vi "Swerve Drive.vi"(0 "X":dbl format="%#_13g", 1 "Z":dbl format="%#_13g", 3 "error in":errorcluster, 5 "Y":dbl format="%#_13g", 6 "Swerve Dev Ref":T3[](array[typedef]), 8 "Drive Dev Ref":T3[](array[typedef]), 9 "Straight Drive":bool, 10 "PigeonIMUDevRef":T1={"DeviceStatus"={"status"=FALSE, "code"=0, "source"=""}, "Device Number"=0, "Type"=352321536, "Device ID"=0, "Handle"=0, "UsageFrame"=0, "Library Path"=path ""} {"Type" items=["CAN"=352321536, "TalonSRX"=33554432]}, 11 "Reverse Drive":bool, 12 "Low Sensitivity":bool, 14 "X Drive":bool, 15 "Field Relative Active":bool) -> (4 "error out":errorcluster)   [LabVIEW 2017, in "Huskie Swerve.lvlib"]
uses:
  Huskie Swerve.lvlib
  <vilib>/Rock Robotics/WPI/MotorControl/WPI_MotorControlDeviceRef.ctl
  <vilib>/Rock Robotics/WPI/MotorControl/WPI_MotorControlType.ctl
  <vilib>/Rock Robotics/SystemInterfaces/DIO/FPGA_DIOPWMChannel.ctl
  <vilib>/Rock Robotics/WPI/PWM/WPI_PWMDeadband.ctl
  <vilib>/Rock Robotics/SystemInterfaces/DIO/FPGA_DIOChannel.ctl
  <vilib>/Rock Robotics/WPI/ThirdParty/Phoenix-LabVIEW/Pigeon IMU/CTRE_PigeonIMU_DeviceRef.ctl
  Public/Documents/Cross The Road Electronics/Phoenix-LabVIEW/Pigeon IMU/CTRE_PigeonIMU_ConnectionType.ctl
  <vilib>/Rock Robotics/WPI/ThirdParty/Phoenix-LabVIEW/Motor Controller/Controls/CTRE_Phoenix_MotorControl_ControlMode.ctl
panel:
  out "Constants":cluster{"a":dbl, "b":dbl, "c":dbl, "d":dbl}[](array[cluster])
  out "Direction":dbl[](array[numeric])
  out "current pos":dbl[](array[numeric])
  out "setpoint":dbl[](array[numeric])
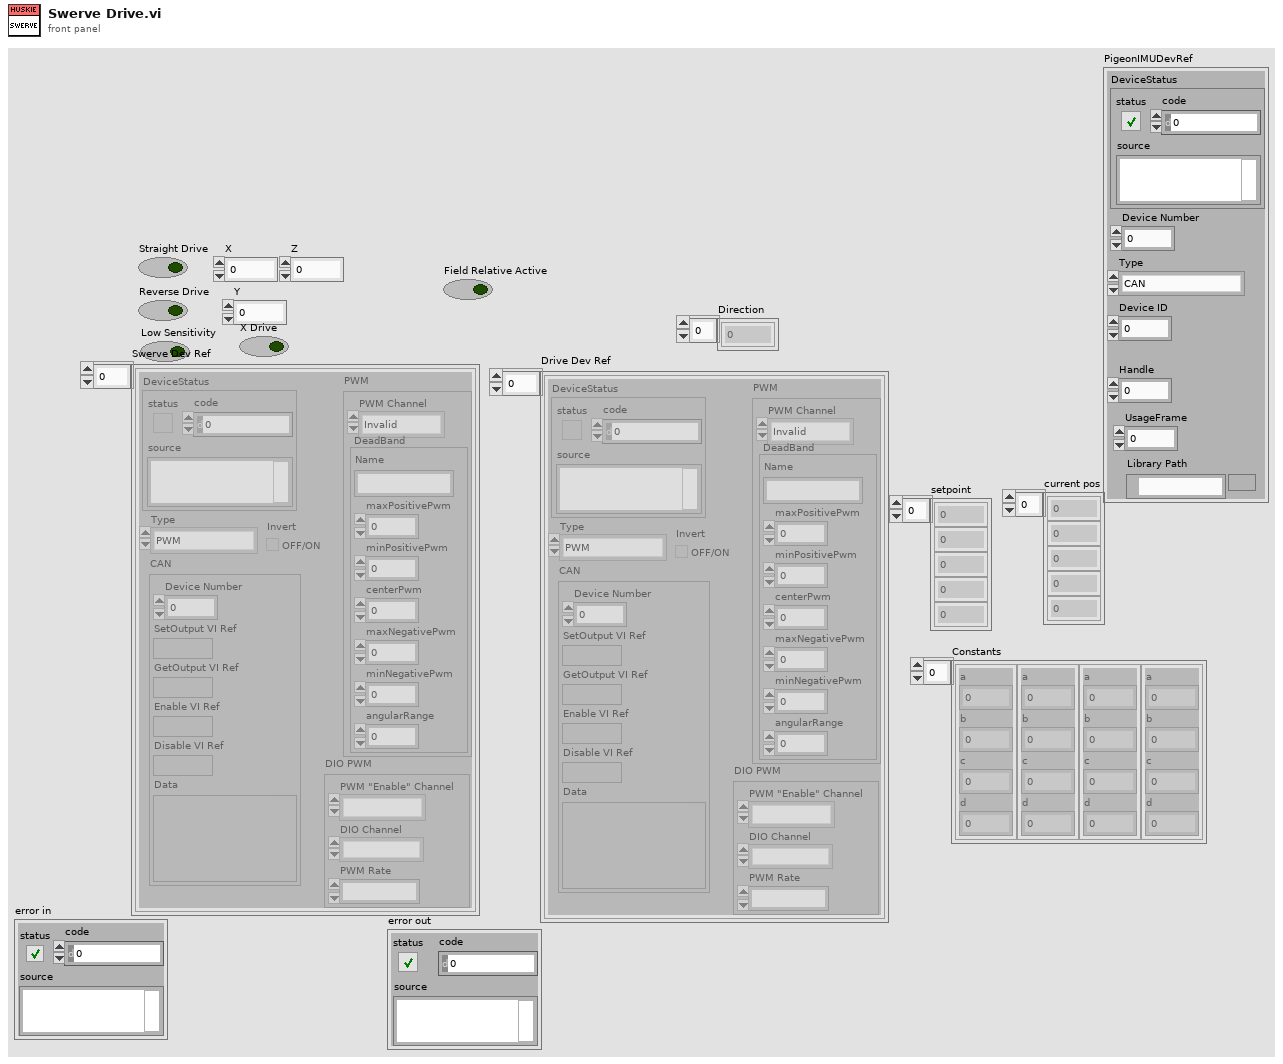
[diagram p1: front panel]
types:
  T1 = typedef "CTRE_PigeonIMU_DeviceRef.ctl" = cluster{"DeviceStatus":errorcluster, "Device Number":u8, "Type":T2, "Device ID":u32, "Handle":u64, "UsageFrame":u32, "Library Path":path}
  T2 = typedef "CTRE_PigeonIMU_ConnectionType.ctl" = u32
  T3 = typedef "WPI_MotorControlDeviceRef.ctl" = cluster{"DeviceStatus":errorcluster, "Type":T4, "PWM":cluster{"PWM Channel":T5, "DeadBand":T6}, "CAN":cluster{"Device Number":u8, "SetOutput VI Ref":variant, "GetOutput VI Ref":variant, "Enable VI Ref":variant, "Disable VI Ref":variant, "Data":variant}, "Invert":bool, "DIO PWM":cluster{"PWM \"Enable\" Channel":T5, "DIOChannel":T7, "PWM Rate":dbl}}
  T4 = typedef "WPI_MotorControlType.ctl" = enum16{"PWM", "CAN", "DIO PWM"}
  T5 = typedef "FPGA_DIOPWMChannel.ctl" = enum8{"PWM 0", "PWM 1", "PWM 2", "PWM 3", "PWM 4", "PWM 5", "PWM 6", "PWM 7", "PWM 8", "PWM 9", "PWM MXP 0", "PWM MXP 1", "PWM MXP 2", "PWM MXP 3", "PWM MXP 4", "PWM MXP 5", "PWM MXP 6", "PWM MXP 7", "PWM MXP 8", "PWM MXP 9", "Invalid"}
  T6 = typedef "WPI_PWMDeadband.ctl" = cluster{"Name":string, "maxPositivePwm":i32, "minPositivePwm":i32, "centerPwm":i32, "maxNegativePwm":i32, "minNegativePwm":i32, "angularRange":u16}
  T7 = typedef "FPGA_DIOChannel.ctl" = enum8{"DIO 0", "DIO 1", "DIO 2", "DIO 3", "DIO 4", "DIO 5", "DIO 6", "DIO 7", "DIO 8", "DIO 9", "DIO MXP 0", "DIO MXP 1", "DIO MXP 2", "DIO MXP 3", "DIO MXP 4", "DIO MXP 5", "DIO MXP 6", "DIO MXP 7", "DIO MXP 8", "DIO MXP 9", "DIO MXP 10", "DIO MXP 11", "DIO MXP 12", "DIO MXP 13", "DIO MXP 14", "DIO MXP 15", "SPI Port CS1", "SPI Port CS2", "SPI Port CS3", "SPI Port MISO", "SPI Port MOSI", "Invalid"}
  T8 = typedef "CTRE_Phoenix_MotorControl_ControlMode.ctl" = u16
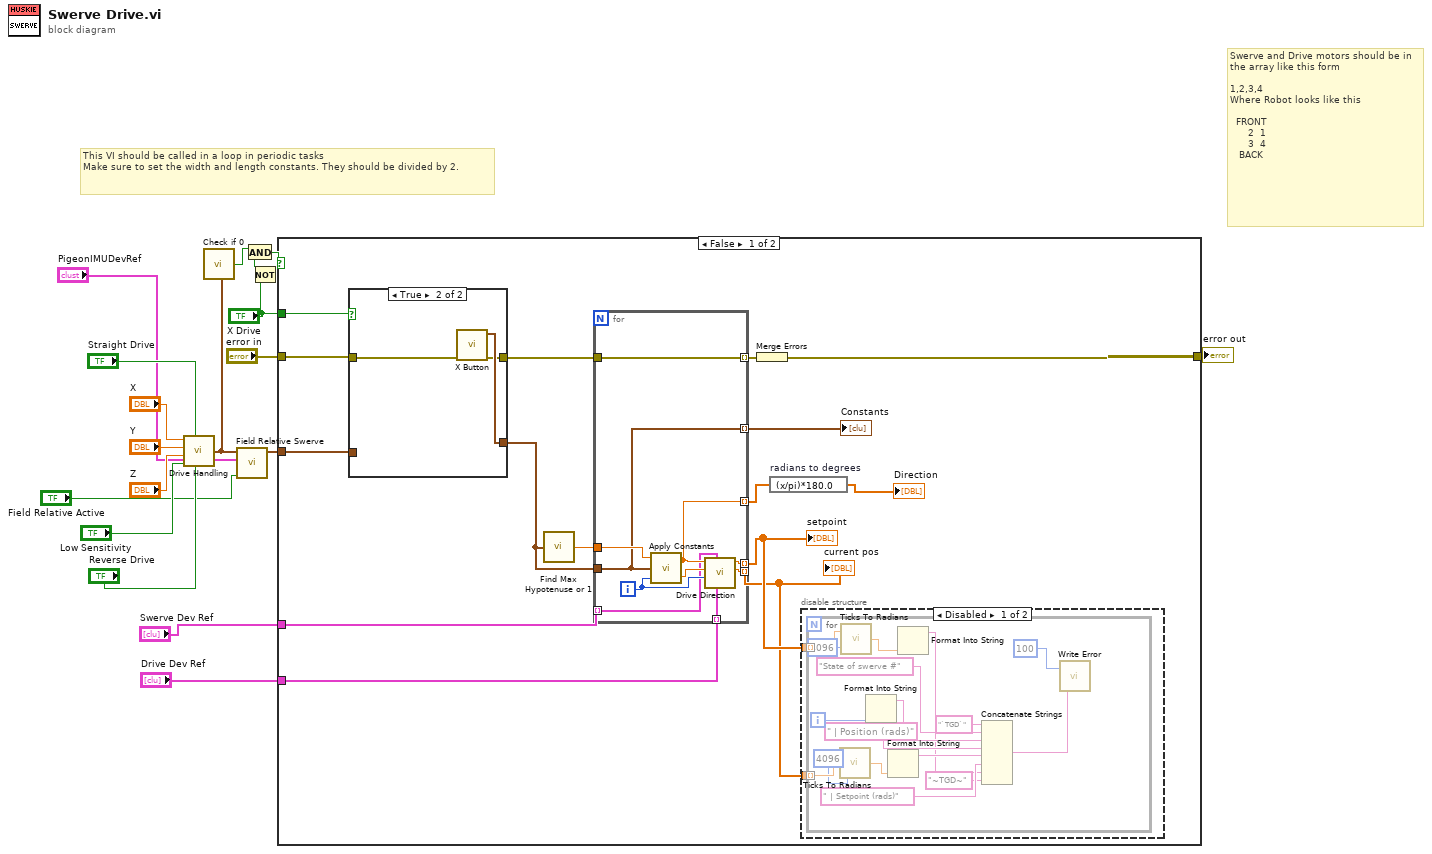
[diagram p0: block diagram]
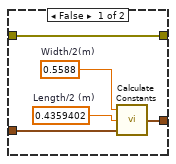
[diagram p3: hidden frame]
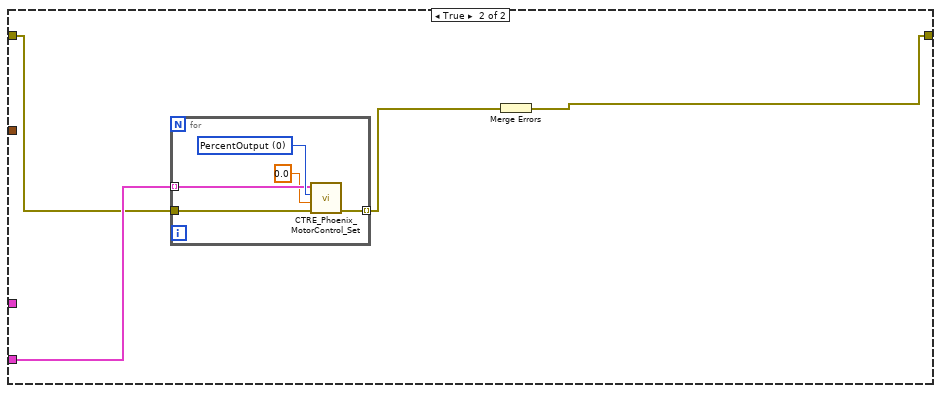
[diagram p4: hidden frame]
diagram:
  # "Swerve and Drive motors should be in the array like this form\n\n1,2,3,4\nWhere Robot looks like this\n\n  FRONT      \n      2  1\n      3  4\n   BACK"
  # "This VI should be called in a loop in periodic tasks\nMake sure to set the width and length constants. They should be divided by 2."
  n1 = call "Drive Handling.vi"("Reverse"="Reverse Drive", "Straight"="Straight Drive", "Low Sensitivity"="Low Sensitivity", "Z"="Z", "Y"="Y", "X"="X") -> ("Axes Magnitudes"=w12:cluster{"X":dbl, "Y":dbl, "Z":dbl})
  n2 = call "Check if 0.vi"("Axes Magnitudes"=w12) -> ("result"=w6:bool)
  n3 = call "Field Relative Swerve.vi"("Field Relative Active"="Field Relative Active", "PigeonIMUDevRef"="PigeonIMUDevRef", "Axes Magnitudes"=w12) -> ("Axes Mag. Changed"=w9:cluster{"X":dbl, "Y":dbl, "Z":dbl})  [unwired: 8 in]
  n4 = Not(x="X Drive") -> (.not. x?=w4:bool)
  n5 = And(x=w6, y=w4) -> (x .and. y?=w7:bool)
  n6 = case shown="False" w7 {
    tunnel: w9 -> [w33 _]
    tunnel: "error in" -> [w27 w73]
    tunnel: [w32 w71] -> w10
    tunnel: "X Drive" -> [w28 _]
    tunnel: "Drive Dev Ref" -> [w22 w74]
    tunnel: "Swerve Dev Ref" -> [w21 _]
    frame False {
      n7 = case shown="True" w28 {
        tunnel: w33 -> [w57 _]
        tunnel: [w55 w60] -> w31
        tunnel: w27 -> [w54 w59]
        tunnel: [w54 w58] -> w26
        frame False {
          w53 = 0.4359402  # Length/2 (m)
          w56 = 0.5588  # Width/2(m)
          n8 = call "Calculate Constants.vi"("Axes Magnitudes"=w57, "Length/2"=w53, "Width/2"=w56) -> ("constants cluster"=w55:cluster{"a":dbl, "b":dbl, "c":dbl, "d":dbl})
        }
        frame True {
          n9 = call "X Button.vi"("error in"=w59) -> ("error out"=w58:errorcluster, "constants cluster"=w60:cluster{"a":dbl, "b":dbl, "c":dbl, "d":dbl})  [unwired: 9 in]
        }
      }
      n10 = call "Find Max Hypotenuse or 1.vi"("constants"=w31) -> ("Max or 1"=w30:dbl)
      n11 = for {
        tunnel: w31 -> [w63]
        tunnel: w30 -> [w70]
        tunnel: [w68] -> w29 mode=indexing
        tunnel: w26 -> [w68]
        tunnel: [w66] -> w20 mode=indexing
        tunnel: [w65] -> w19 mode=indexing
        tunnel: [w64] -> w25 mode=indexing
        tunnel: [w63] -> w23 mode=indexing
        tunnel: w22 -> [w62] mode=indexing
        tunnel: w21 -> [w61] mode=indexing
        i -> [w67]
        n12 = call "Apply Constants.vi"("Module Number"=w67, "constants cluster"=w63, "Max Speed or 1"=w70) -> ("Magnitude"=w69:dbl, "Desired Direction (rad)"=w64:dbl)
        n13 = call "Drive Direction.vi"("Drive DevRef"=w62, "Swerve DevRef"=w61, "Module Number"=w67, "Wheel Power"=w69, "Desired direction (radians)"=w64) -> ("Sensor Position"=w65:dbl, "setpoint"=w66:dbl)  [unwired: 5 in]
      }
      "setpoint" <- w20
      "current pos" <- w19
      "Constants" <- w23
      n14 = Merge Errors(w29) -> (w32:errorcluster)
      n15 = expression code="(x/pi)*180.0" "radians to degrees"(w25) -> (→"Direction":dbl[])
      n16 = disable-structure shown="Disabled" {
        disable-tunnel: w20 -> [w35 _]
        disable-tunnel: w19 -> [w34 _]
        frame Disabled {
          n17 = for {
            tunnel: w35 -> [w41] mode=indexing
            tunnel: w34 -> [w43] mode=indexing
            i -> [w49]
            n18 = call "Ticks To Radians.vi"("Ticks/Rev"=4096, "Ticks"=w43) -> ("Radians"=w44:dbl)
            n19 = call "Ticks To Radians.vi"("Ticks/Rev"=4096, "Ticks"=w41) -> ("Radians"=w39:dbl)
            n20 = Format Into String(w49) -> (resulting string=w48:string)  [unwired: 3 in, 1 out]
            n21 = Format Into String(w44) -> (resulting string=w45:string)  [unwired: 3 in, 1 out]
            n22 = Format Into String(w39) -> (resulting string=w38:string)  [unwired: 3 in, 1 out]
            n23 = Concatenate Strings("`TGD`" ("string"), "State of swerve #", w48, " | Position (rads)", w45, " | Setpoint (rads)", w38, "~TGD~" ("string")) -> (w52:string)
            n24 = call "Write Error.vi"("Message To Write"=w52, "Error Code"=100) -> ()  [unwired: 1 out]
          }
        }
        frame Enabled {
        }
      }
    }
    frame True {
      n25 = for {
        tunnel: w74 -> [w78] mode=indexing
        tunnel: w73 -> [w76]
        tunnel: [w75] -> w72 mode=indexing
        w79 = T8 0 items=["PercentOutput"=0, "Position"=1, "Velocity"=2, "Current"=3, "Follower"=5, "MotionProfile"=6, "MotionMagic"=7, "MotionMagicArc"=8, "MotionProfileArc"=10, "Disabled"=15] ("Control Mode")
        n26 = call "CTRE_Phoenix_MotorControl_Set.vi"("error in (no error)"=w76, "Output"=0.0, "Control Mode"=w79, "PhoenixMotorControlDevRef"=w78) -> ("error out"=w75:errorcluster)  [unwired: 6 in, 1 out]
      }
      n27 = Merge Errors(w72) -> (w71:errorcluster)
    }
  }
  "error out" <- w10
